vi "Error Query.vi"(8 "error in (no error)":errorcluster, 11 "VISA resource name":refnum<visa-resource-name>) -> (0 "error out":errorcluster, 1 "Error Message":string, 2 "Error Code":i32[](array[numeric]), 3 "VISA resource name out":refnum<visa-resource-name>)   [LabVIEW 2017, in "ADCMT7351_ADC.lvlib"]
doc: "Queries the instrument for any errors in the instrument's error queue. It will continue to read errors until all errors have been read from the instrument. Any errors will be returned in the <B>error out</B> control.\n\n<B>Note:</B>\nThis VI is called automatically by most driver VIs so it is not usually necessary to call this in an application."
uses:
  ADCMT7351_ADC.lvlib
  Instance           1 19Saved   Error Query .vi
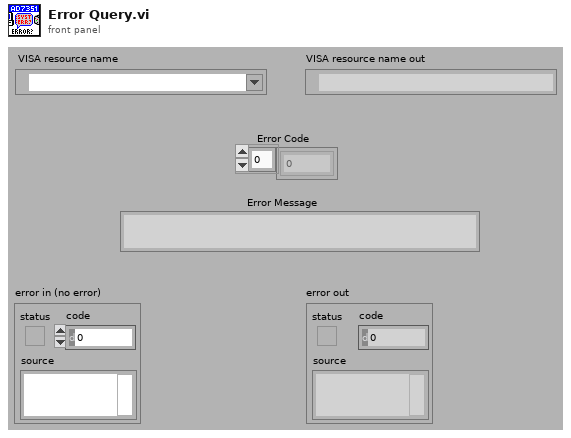
[diagram p1: front panel]
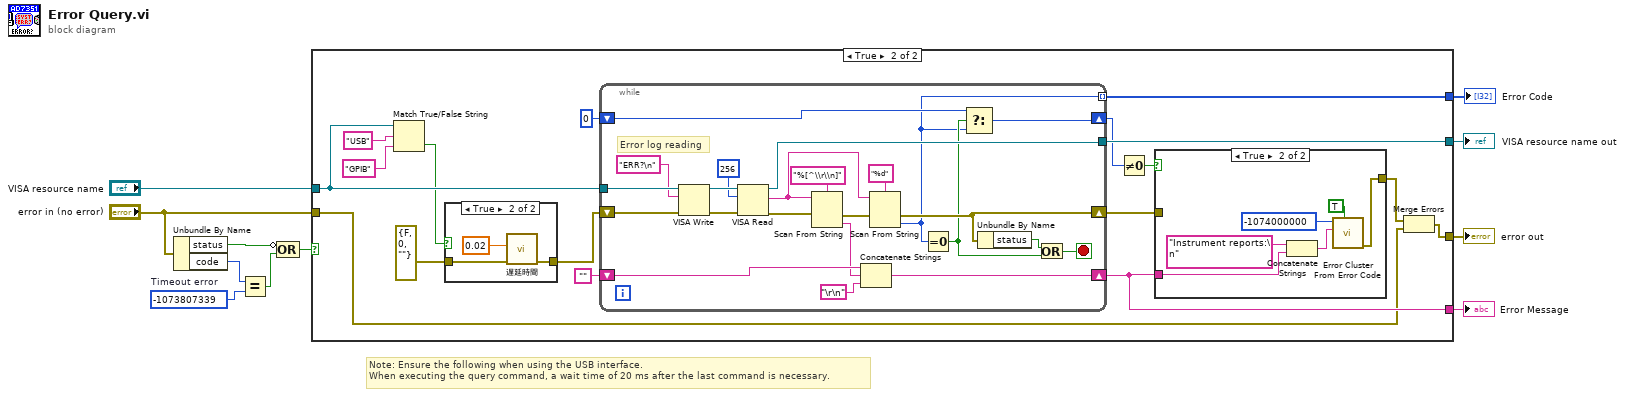
[diagram p0: block diagram]
diagram:
  w6 = -1073807339  # Timeout error
  # "Note: Ensure the following when using the USB interface.\nWhen executing the query command, a wait time of 20 ms after the last command is necessary."
  n1 = Unbundle By Name("error in (no error)") -> ("status"=w7:bool, "code"=w4:i32)
  n2 = Equal?(x=w4, y=w6) -> (x = y?=w5:bool)
  n3 = Compound Arithmetic op=OR(invert w7, w5) -> (w3:bool)
  n4 = case shown="True" w3 {
    tunnel: [w15 w32] -> w11
    tunnel: "VISA resource name" -> [w15 w18]
    tunnel: "error in (no error)" -> [w14 w23]
    tunnel: [w14 w30] -> w9
    tunnel: ["" w25] -> w2
    tunnel: [i32[] [] w24] -> w1
    frame False {
    }
    frame True {
      n5 = Match True/False String(2:"GPIB" ("false文字列"), 3:"USB" ("true文字列"), 4:w18) -> (0:w16:bool)  [unwired: 1 out]
      n6 = case shown="True" w16 {
        tunnel: [w33 w35] -> w21
        tunnel: errorcluster {"status"=FALSE, "code"=0, "source"=""} ("error in (no error)") -> [w33 w34]
        frame False {
        }
        frame True {
          n7 = call "遅延時間"("error in (no error)"=w34, "Delay Time (s)"=0.02) -> ("error out"=w35:errorcluster)  [unwired: 9 in]
        }
      }
      n8 = while {
        tunnel: [w66] -> w32
        tunnel: w18 -> [w65]
        shift-right: [w55] -> w25
        shift-left: "" -> [w58]
        shift-right: [w53] -> w26
        shift-left: 0 -> [w54]
        shift-right: [w52] -> w22
        shift-left: w21 -> [w45]
        tunnel: [w47] -> w24 mode=indexing
        stop <- w46 stop-if-true
        # "Error log reading"
        n9 = VISA Write(VISA resource name=w65, write buffer="ERR?\n" ("Error Query Command"), error in (no error)=w45) -> (VISA resource name out=w64:refnum<visa-resource-name>, error out=w62:errorcluster)  [unwired: 1 out]
        n10 = VISA Read(VISA resource name=w64, byte count=u32 256 ("Bytes"), error in (no error)=w62) -> (VISA resource name out=w66:refnum<visa-resource-name>, read buffer=w59:string, error out=w51:errorcluster)  [unwired: 1 out]
        n11 = Scan From String(format string="%[^\\r\\n]", input string=w59, error in=w51) -> (error out=w50:errorcluster, output 1=w56:string)  [unwired: 2 in, 2 out]
        n12 = Concatenate Strings(w58, w56, "\r\n") -> (w55:string)
        n13 = Scan From String(format string="%d", input string=w59, error in=w50) -> (error out=w52:errorcluster, output 1=w47:i32)  [unwired: 2 in, 2 out]
        n14 = Equal To 0?(x=w47) -> (x = 0?=w48:bool)
        n15 = Select(t=w54, s=w48, f=w47) -> (s? t:f=w53:i32)
        n16 = Unbundle By Name(w52) -> ("status"=w49:bool)
        n17 = Or(x=w49, y=w48) -> (x .or. y?=w46:bool)
      }
      n18 = Not Equal To 0?(x=w26) -> (x != 0?=w28:bool)
      n19 = case shown="True" w28 {
        tunnel: w25 -> [_ w42]
        tunnel: [w37 w38] -> w27
        tunnel: w22 -> [w37 _]
        frame False {
        }
        frame True {
          n20 = Concatenate Strings("Instrument reports:\n" ("Source"), w42) -> (w39:string)
          n21 = call <vilib>:"Error Cluster From Error Code.vi"("show call chain? (False)"=TRUE, "error message (\"\")"=w39, "error code (0)"=-1074000000 ("Code")) -> ("error out"=w38:errorcluster)  [unwired: 6 in]
        }
      }
      n22 = Merge Errors(w27, w23) -> (w30:errorcluster)
    }
  }
  "VISA resource name out" <- w11
  "error out" <- w9
  "Error Message" <- w2
  "Error Code" <- w1
